vi "GenTargetSquat.vi"() -> ()   [LabVIEW 2016]
uses:
  Classes/CAlex2/TypeDef/CAlexVersion.ctl
  Sim&Process/DataProcess/CAlex2-Data/CAlex2_Data.lvclass
  C:/Users/Rand/Desktop/Bilateral-controller/CAlex2-controller/Sim&Process/DataProcess/ExpData/ExpData.lvclass
  Sim&Process/DataProcess/CAlex2-Data/PropertyNodes/Get_JointAngles.vi
  <vilib>/Utility/file.llb/Write Delimited Spreadsheet (string).vi
  <vilib>/Utility/file.llb/Write Delimited Spreadsheet (DBL).vi
  Sim&Process/DataProcess/ExpData/ExpData.lvclass
  <vilib>/AuZn/auzn custom VIs/AuZnCustomVI.lvlib
  Classes/CAlex2/CAlex2.lvclass
panel:
  out "TargetTraj 2":dbl[][](array[numeric])
  out "Xmin":dbl
  out "Xmax":dbl
  out "Ymin":dbl
  out "Ymax":dbl
  out "CAlexVersion":T1=enum."Mobile"
  out "AveragedJointAngle":dbl[][](array[numeric])
  out "TargetJointAngle":dbl[][](array[numeric])
  out "TargetTraj":dbl[][](array[numeric])
  in  "Save":bool
  in  "Ankle Flex":dbl=1.0 format="%#_13g"
  out "Leg Length":cluster{"Thigh":dbl, "Shank":dbl}
  in  "Scale Method":enum16{"Squat Depth", "Squat Angles"}(ring)
  in  "OutputLength":i32=500
  in  "Depth/Adduct":dbl=1.3 format="%#_13g"
  out "Array":dbl[](array[numeric])
  in  "Update":bool
  in  "Open":bool
  in  "stop":bool
  in  "EndTime":dbl=240.0
  in  "StartTime":dbl=60.0
  in  "Cut":bool
  out "AveragedTrajectory":dbl[][](graph)
  out "Averaged":cluster{"Mean":dbl[], "Mean":dbl[]}[](graph)
  out "Stacked":T2(graph)
  out "Ankle - X":dbl[][](graph)
  in  "Cut Parameter":dbl=100.0
  in  "Path":path=path "C:/Users/Rand/Desktop/squat simulated.txt"
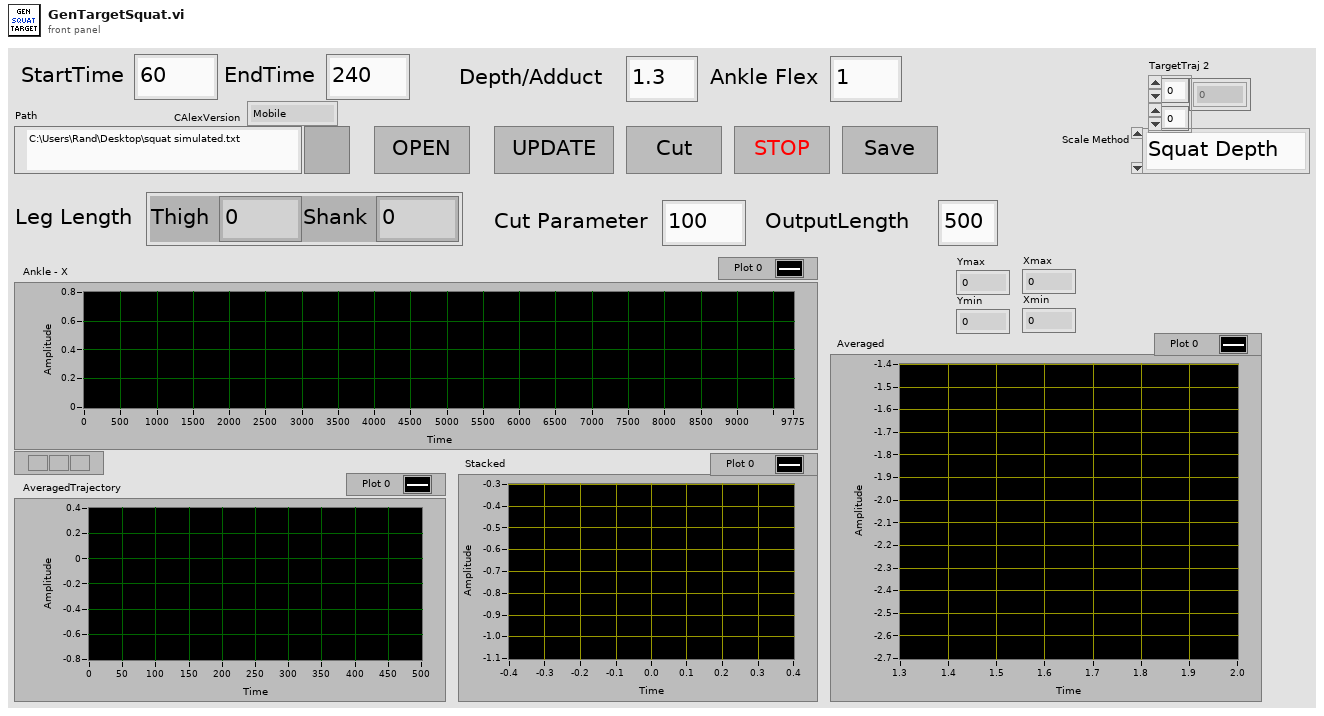
[diagram p1: front panel]
types:
  T1 = typedef "CAlex2.lvclass/CAlexVersion.ctl" = enum16{"Bilateral_Squat", "Squat", "Treadmill", "Mobile"}
  T2 = cluster{"DataAccess:WaistPosition":dbl[], "DataAccess:WaistPosition":dbl[]}
  T3 = enum16{"open", "replace", "create", "open or create", "replace or create", "replace or create with confirmation"}
  T4 = cluster{"ThighLt":dbl, "ShankLt":dbl, "HipWd":dbl}
  T5 = cluster{"ScaledJointAngles":dbl[], "ScaledJointAngles":dbl[]}
  T6 = cluster{"ScaledJointAngles":dbl[], "ScaledJointAngles":dbl[]}[]
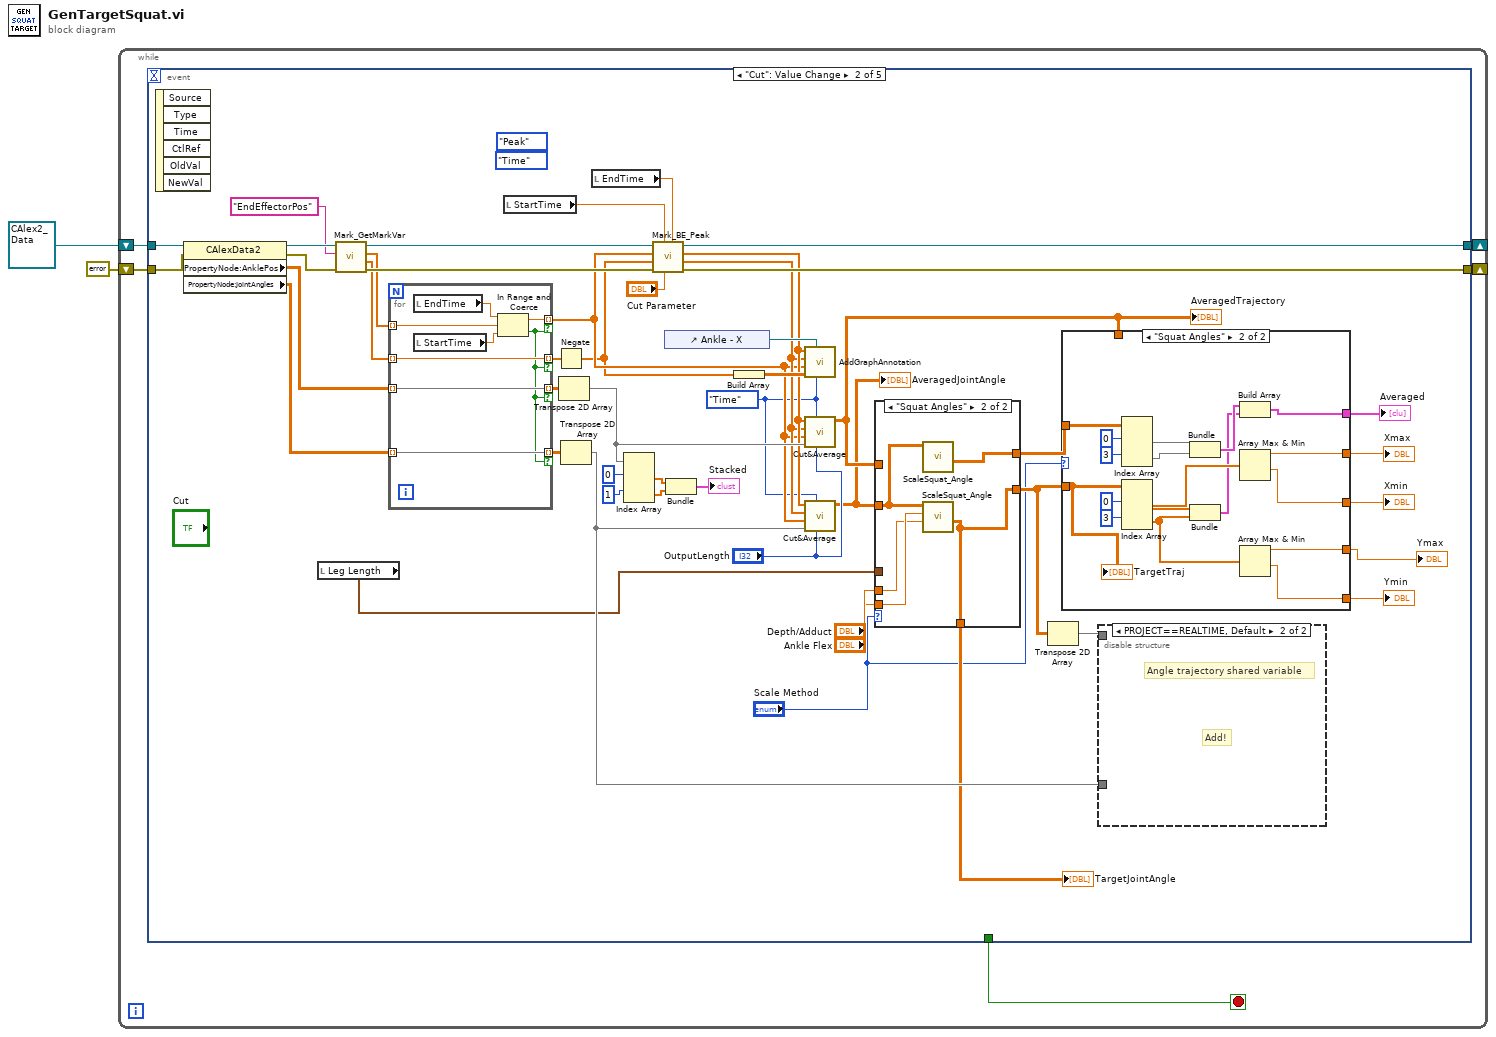
[diagram p0: block diagram]
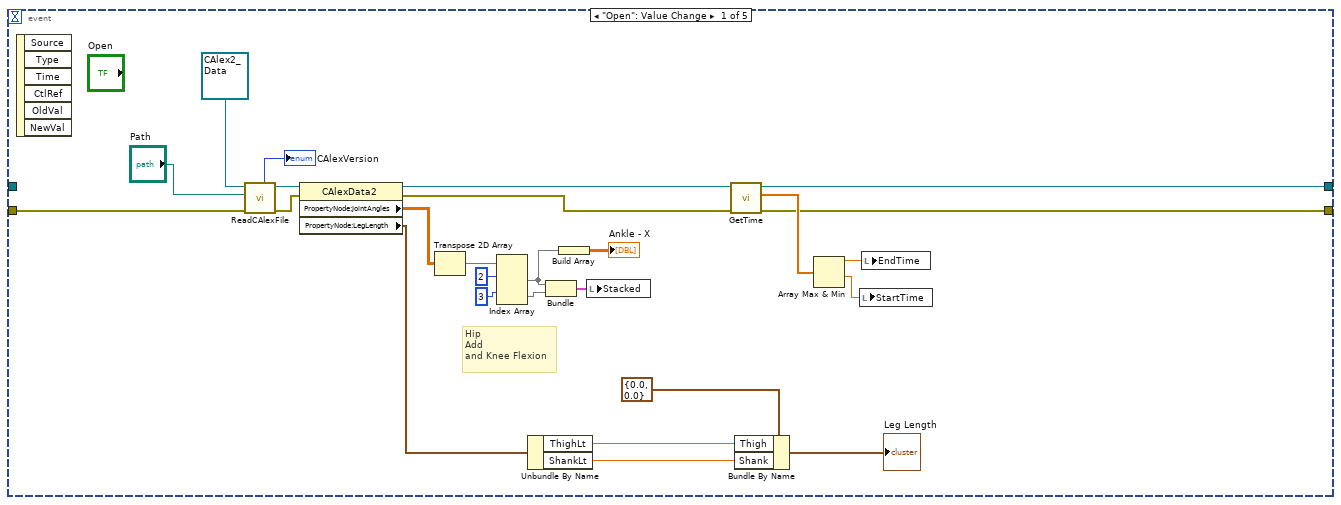
[diagram p2: hidden frame]
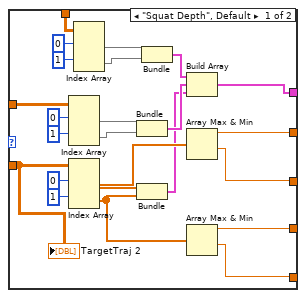
[diagram p3: hidden frame]
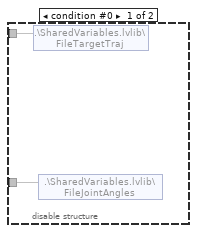
[diagram p4: hidden frame]
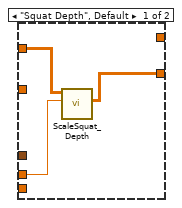
[diagram p5: hidden frame]
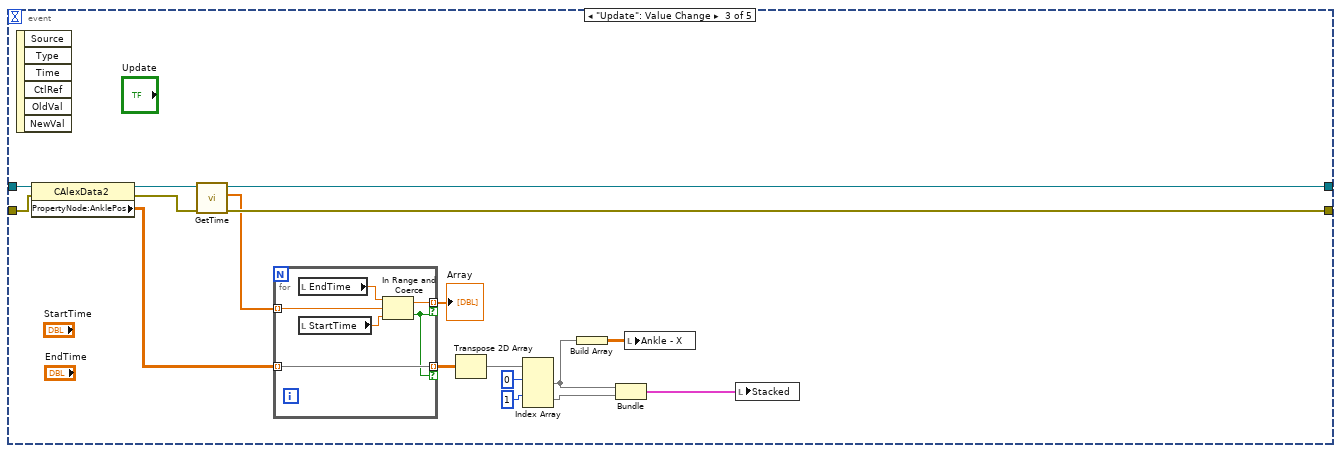
[diagram p6: hidden frame]
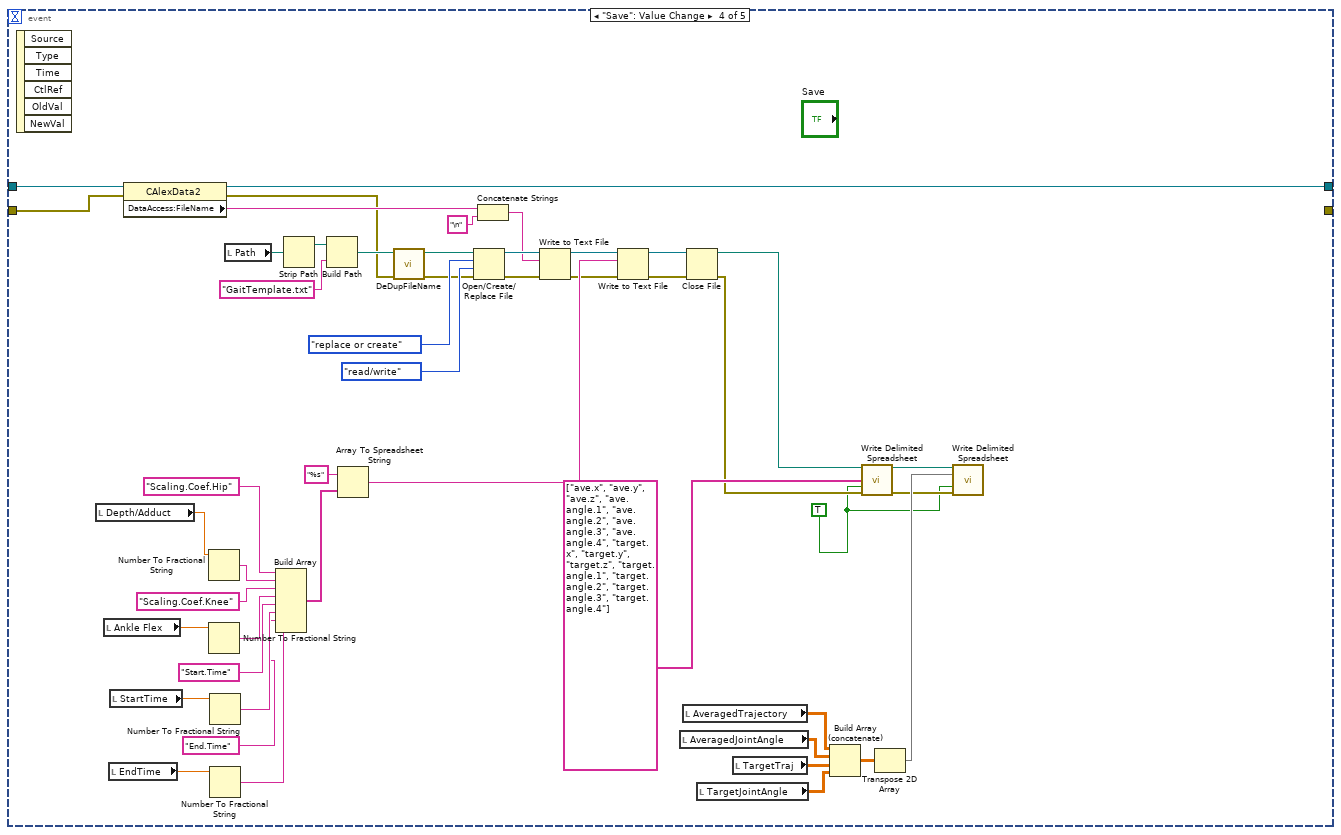
[diagram p7: hidden frame]
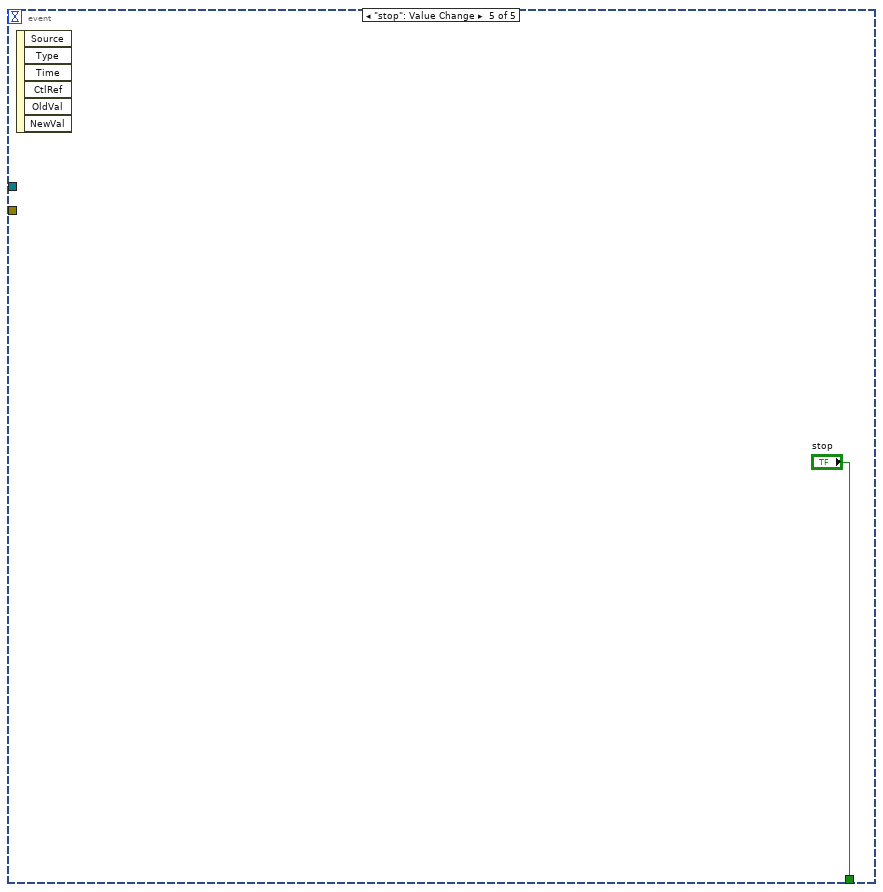
[diagram p8: hidden frame]
diagram:
  n1 = while {
    shift-right: [w4] -> _
    shift-left: refnum<class "CAlex2_Data.lvclass"> refnum ("CAlexData") -> [w7]
    shift-right: [w5] -> _
    shift-left: errorcluster {"status"=FALSE, "code"=0, "source"=""} ("error out") -> [w6]
    stop <- w3 stop-if-true
    n2 = event shown="[1] \"Cut\": Value Change" {
      selector: _ -> [_ _ _ _ _]
      dyn-events: _ -> [_ _ _ _ _]
      timeout: _ -> [_ _ _ _ _]
      tunnel: w7 -> [_ w74 w154 w176 _]
      tunnel: w6 -> [w23 w72 w153 w177 _]
      tunnel: [w20 w64 w145 _ _] -> w5
      tunnel: [w22 w63 w147 w175 _] -> w4
      tunnel: [_ _ _ _ "stop"] -> w3
      event "Open": Value Change {
        # "Hip\nAdd\nand Knee Flexion"
        n3 = event-data() -> ()  [unwired: 1 in, 6 out]
        n4 = call "ReadCAlexFile.vi"("error in (no error)"=w23, "ExpData File Path"="Path", "CAlexData2"=refnum<class "CAlex2_Data.lvclass"> refnum ("CAlexData")) -> ("error out"=w17:errorcluster, "CAlexData 2"=w19:refnum<class "CAlex2_Data.lvclass">, "CAlexVersion"=→"CAlexVersion":T1)  [unwired: 6 in]
        n5 = property class="CAlexData2"(reference=w19, error in=w17) -> (reference out=w18:refnum<class "CAlex2_Data.lvclass">, error out=w16:errorcluster, "PropertyNode:JointAngles"=w15:dbl[][], "PropertyNode:LegLength"=w14:T4)
        n6 = Transpose 2D Array(2D array=w15) -> (transposed array=w9:dbl[][])
        n7 = Index Array(array=w9, index (row) #1=2 ("index (row)"), index (row) #2=3 ("index (row)")) -> (element #1=w27:dbl[], element #2=w26:dbl[])  [unwired: 2 in]
        n8 = Unbundle By Name(w14) -> ("ThighLt"=w12:dbl, "ShankLt"=w11:dbl)
        n9 = Bundle(w27, w26) -> (w29:cluster{dbl[], dbl[]})  [unwired: 1 in]
        n10 = Build Array(w27) -> (→"Ankle - X":dbl[][])
        n11 = local write "Stacked"(w29) -> ()
        n12 = call "GetTime.vi"("error in (no error)"=w16, "ExpData in"=w18) -> ("error out"=w20:errorcluster, "Time"=w21:dbl[], "ExpData out"=w22:refnum<class "CAlex2_Data.lvclass">)  [unwired: 7 in]
        n13 = Bundle By Name(cluster=cluster{"Thigh":dbl, "Shank":dbl} {"Thigh"=0.0, "Shank"=0.0} ("Leg Length"), "Thigh"=w12, "Shank"=w11) -> (→"Leg Length":cluster{"Thigh":dbl, "Shank":dbl})
        n14 = Array Max & Min(array=w21) -> (max value=w33:dbl, min value=w32:dbl)  [unwired: 2 out]
        n15 = local write "StartTime"(w32) -> ()
        n16 = local write "EndTime"(w33) -> ()
      }
      event "Cut": Value Change {
        w57 = enum16{"Time", "Percentage", "Index"}."Time" ("Input Type")
        (unwired) enum16{"Peak", "Valley"}."Peak" ("Peak/Valley")
        (unwired) enum16{"Time", "Percentage", "Index"}."Time" ("Output Type")
        n17 = event-data() -> ()  [unwired: 1 in, 6 out]
        n18 = property class="CAlexData2"(reference=w74, error in=w72) -> (reference out=w73:refnum<class "CAlex2_Data.lvclass">, error out=w71:errorcluster, "PropertyNode:AnklePos"=w45:dbl[][], "PropertyNode:JointAngles"=w44:dbl[][])
        n19 = local read "Leg Length"() -> (w47:cluster{"Thigh":dbl, "Shank":dbl})
        n20 = call "Mark_GetMarkVar.vi"("error in (no error)"=w71, "VarName"="EndEffectorPos", "ExpData in"=w73) -> ("error out"=w81:errorcluster, "MarkVar"=w79:dbl[], "Time"=w80:dbl[], "ExpData out"=w75:refnum<class "CAlex2_Data.lvclass">)  [unwired: 3 in, 2 out]
        n21 = for {
          tunnel: w80 -> [w140] mode=indexing
          tunnel: w79 -> [w136] mode=indexing
          tunnel: [w137] -> w59 mode=indexing if=w133
          tunnel: [w136] -> w78 mode=indexing if=w133
          tunnel: w45 -> [w135] mode=indexing
          tunnel: [w135] -> w70 mode=indexing if=w133
          tunnel: w44 -> [w134] mode=indexing
          tunnel: [w134] -> w56 mode=indexing if=w133
          n22 = local read "EndTime"() -> (w138:dbl)
          n23 = local read "StartTime"() -> (w139:dbl)
          n24 = In Range and Coerce(upper limit=w138, x=w140, lower limit=w139) -> (coerced(x)=w137:dbl, In Range?=w133:bool)
        }
        n25 = local read "StartTime"() -> (w42:dbl)
        n26 = Negate(x=w78) -> (-x=w41:dbl[])
        n27 = Transpose 2D Array(2D array=w70) -> (transposed array=w62:dbl[][])
        n28 = Transpose 2D Array(2D array=w56) -> (transposed array=w51:dbl[][])
        n29 = local read "EndTime"() -> (w43:dbl)
        n30 = Index Array(array=w62, index (row) #1=0 ("index (row)"), index (row) #2=1 ("index (row)")) -> (element #1=w67:dbl[], element #2=w66:dbl[])  [unwired: 2 in]
        n31 = call "Mark_BE_Peak.vi"("End Time"=w43, "HalfWidth"="Cut Parameter", "Start Time"=w42, "error in (no error)"=w81, "Input"=w41, "Time"=w59, "CarexData In"=w75) -> ("error out"=w64:errorcluster, "End"=w60:dbl[], "Begin"=w61:dbl[], "CarexData Out"=w63:refnum<class "CAlex2_Data.lvclass">)  [unwired: 1 in]
        n32 = control-ref of="Ankle - X"() -> (w76:refnum<vi>)
        n33 = Bundle(w67, w66) -> (→"Stacked":cluster{dbl[], dbl[]})  [unwired: 1 in]
        n34 = Build Array(w41) -> (w77:dbl[][])
        n35 = call <vilib>:"AddGraphAnnotation.vi"("Input Type (Time)"=w57, "WaveformGraph in"=w76, "Array"=w77, "Time"=w59, "Valleys  (Yellow)"=w60, "Peaks (Red)"=w61) -> ()  [unwired: 4 in, 2 out]
        n36 = call <vilib>:"Cut&Average.vi"("Dilate Length (200)"="OutputLength", "Input Type (Time)"=w57, "Data"=w62, "Time"=w59, "End"=w60, "Begin"=w61) -> ("Mean"=w54:dbl[][])  [unwired: 5 out]
        "AveragedTrajectory" <- w54
        n37 = call <vilib>:"Cut&Average.vi"("Dilate Length (200)"="OutputLength", "Input Type (Time)"=w57, "Data"=w51, "Time"=w59, "End"=w60, "Begin"=w61) -> ("Mean"=w50:dbl[][])  [unwired: 5 out]
        "AveragedJointAngle" <- w50
        n38 = case shown="\"Squat Angles\"" "Scale Method" {
          tunnel: [w126 w130] -> w52
          tunnel: w50 -> [_ w132]
          tunnel: w47 -> [_ _]
          tunnel: "Depth/Adduct" -> [w127 w128]
          tunnel: w54 -> [w125 _]
          tunnel: "Ankle Flex" -> [_ w129]
          tunnel: [_ w130] -> w49
          tunnel: [_ w131] -> w48
          frame "Squat Depth", Default {
            n39 = call "ScaleSquat_Depth.vi"("ScalingCoef"=w127, "Averaged Squat Trajectory"=w125) -> ("ScaledGait"=w126:dbl[][])  [unwired: 8 in, 1 out]
          }
          frame "Squat Angles" {
            n40 = call "ScaleSquat_Angle.vi"("AverageJointAngles"=w132) -> ("ScaledJointAngles"=w131:dbl[][])  [unwired: 10 in]
            n41 = call "ScaleSquat_Angle.vi"("ScalingCoef Hip Add"=w128, "ScalingCoef Ankle Flex"=w129, "AverageJointAngles"=w132) -> ("ScaledJointAngles"=w130:dbl[][])  [unwired: 8 in]
          }
        }
        "TargetJointAngle" <- w49
        n42 = Transpose 2D Array(2D array=w52) -> (transposed array=w40:dbl[][])
        n43 = case shown="\"Squat Angles\"" "Scale Method" {
          tunnel: w54 -> [w99 _]
          tunnel: w52 -> [w98 w120]
          tunnel: w48 -> [w93 w115]
          tunnel: [w84 w110] -> w38
          tunnel: [w85 w109] -> w37
          tunnel: [w86 w108] -> w34
          tunnel: [w87 w107] -> w36
          tunnel: [w83 w106] -> w35
          frame "Squat Depth", Default {
            n44 = Index Array(array=w93, index (row) #1=0 ("index (row)"), index (row) #2=1 ("index (row)")) -> (element #1=w95:dbl[], element #2=w94:dbl[])  [unwired: 2 in]
            n45 = Index Array(array=w98, index (row) #1=0 ("index (row)"), index (row) #2=1 ("index (row)")) -> (element #1=w89:dbl[], element #2=w90:dbl[])  [unwired: 2 in]
            n46 = Index Array(array=w99, index (row) #1=0 ("index (row)"), index (row) #2=1 ("index (row)")) -> (element #1=w102:dbl[], element #2=w103:dbl[])  [unwired: 2 in]
            n47 = Bundle("ScaledJointAngles"=w95, "ScaledJointAngles"=w94) -> (w91:T5)  [unwired: 1 in]
            n48 = Bundle("ScaledJointAngles"=w89, "ScaledJointAngles"=w90) -> (w88:T5)  [unwired: 1 in]
            n49 = Bundle("Mean"=w102, "Mean"=w103) -> (w92:cluster{"Mean":dbl[], "Mean":dbl[]})  [unwired: 1 in]
            n50 = Build Array(w92, w91, w88) -> (w83:T6)
            n51 = Array Max & Min(array=w89) -> (max value=w84:dbl, min value=w85:dbl)  [unwired: 2 out]
            n52 = Array Max & Min(array=w90) -> (max value=w86:dbl, min value=w87:dbl)  [unwired: 2 out]
            "TargetTraj 2" <- w98
          }
          frame "Squat Angles" {
            n53 = Index Array(array=w115, index (row) #1=0 ("index (row)"), index (row) #2=3 ("index (row)")) -> (element #1=w117:dbl[], element #2=w116:dbl[])  [unwired: 2 in]
            n54 = Index Array(array=w120, index (row) #1=0 ("index (row)"), index (row) #2=3 ("index (row)")) -> (element #1=w112:dbl[], element #2=w113:dbl[])  [unwired: 2 in]
            n55 = Bundle("ScaledJointAngles"=w117, "ScaledJointAngles"=w116) -> (w114:T5)  [unwired: 1 in]
            n56 = Bundle("ScaledJointAngles"=w112, "ScaledJointAngles"=w113) -> (w111:T5)  [unwired: 1 in]
            n57 = Build Array(w114, w111) -> (w106:T6)
            n58 = Array Max & Min(array=w112) -> (max value=w110:dbl, min value=w109:dbl)  [unwired: 2 out]
            n59 = Array Max & Min(array=w113) -> (max value=w108:dbl, min value=w107:dbl)  [unwired: 2 out]
            "TargetTraj" <- w120
          }
        }
        "Ymax" <- w34
        "Ymin" <- w36
        "Xmax" <- w38
        "Xmin" <- w37
        "Averaged" <- w35
        n60 = disable-structure shown="PROJECT==REALTIME, Default" {
          disable-tunnel: w40 -> [w124 _]
          disable-tunnel: w51 -> [w123 _]
          frame condition #0 {
            n61 = shared-variable ".\\SharedVariables.lvlib\\FileTargetTraj"(w124) -> ()  [unwired: 1 in, 1 out]
            n62 = shared-variable ".\\SharedVariables.lvlib\\FileJointAngles"(w123) -> ()  [unwired: 1 in, 1 out]
          }
          frame condition #1 (active) {
            # "Add!"
            # "Angle trajectory shared variable"
          }
        }
      }
      event "Update": Value Change {
        n63 = event-data() -> ()  [unwired: 1 in, 6 out]
        n64 = property class="CAlexData2"(reference=w154, error in=w153) -> (reference out=w148:refnum<class "CAlex2_Data.lvclass">, error out=w146:errorcluster, "PropertyNode:AnklePos"=w143:dbl[][])
        n65 = call "GetTime.vi"("error in (no error)"=w146, "ExpData in"=w148) -> ("error out"=w145:errorcluster, "Time"=w144:dbl[], "ExpData out"=w147:refnum<class "CAlex2_Data.lvclass">)  [unwired: 7 in]
        n66 = for {
          tunnel: w144 -> [w163] mode=indexing
          tunnel: [w160] -> w152 mode=indexing if=w158
          tunnel: w143 -> [w159] mode=indexing
          tunnel: [w159] -> w142 mode=indexing if=w158
          n67 = local read "EndTime"() -> (w161:dbl)
          n68 = local read "StartTime"() -> (w162:dbl)
          n69 = In Range and Coerce(upper limit=w161, x=w163, lower limit=w162) -> (coerced(x)=w160:dbl, In Range?=w158:bool)
        }
        "Array" <- w152
        n70 = Transpose 2D Array(2D array=w142) -> (transposed array=w141:dbl[][])
        n71 = Index Array(array=w141, index (row) #1=0 ("index (row)"), index (row) #2=1 ("index (row)")) -> (element #1=w150:dbl[], element #2=w149:dbl[])  [unwired: 2 in]
        n72 = Build Array(w150) -> (w151:dbl[][])
        n73 = Bundle(w150, w149) -> (w155:cluster{dbl[], dbl[]})  [unwired: 1 in]
        n74 = local write "Ankle - X"(w151) -> ()
        n75 = local write "Stacked"(w155) -> ()
      }
      event "Save": Value Change {
        w164 = TRUE ("append to file? (new file:F)")
        n76 = event-data() -> ()  [unwired: 1 in, 6 out]
        n77 = local read "Depth/Adduct"() -> (w203:dbl)
        n78 = local read "Ankle Flex"() -> (w202:dbl)
        n79 = local read "EndTime"() -> (w187:dbl)
        n80 = local read "StartTime"() -> (w186:dbl)
        n81 = property class="CAlexData2"(reference=w176, error in=w177) -> (reference out=w175:refnum<class "CAlex2_Data.lvclass">, error out=w165:errorcluster, "DataAccess:FileName"=w174:string)
        n82 = Number To Fractional String(number=w203) -> (F-format string=w200:string)  [unwired: 3 in]
        n83 = Number To Fractional String(number=w202) -> (F-format string=w198:string)  [unwired: 3 in]
        n84 = Number To Fractional String(number=w186) -> (F-format string=w184:string)  [unwired: 3 in]
        n85 = Number To Fractional String(number=w187) -> (F-format string=w182:string)  [unwired: 3 in]
        n86 = local read "Path"() -> (w211:path)
        n87 = Build Array("Scaling.Coef.Hip" ("name or relative path"), w200, "Scaling.Coef.Knee" ("name or relative path"), w198, "Start.Time" ("name or relative path"), w184, "End.Time" ("name or relative path"), w182) -> (w197:string[])
        n88 = Strip Path(path=w211) -> (stripped path=w209:path)  [unwired: 1 out]
        n89 = Build Path(base path=w209, name or relative path="GaitTemplate.txt") -> (appended path=w168:path)
        n90 = Array To Spreadsheet String(array=w197, 3:"%s" ("format string")) -> (spreadsheet string=w196:string)  [unwired: 1 in]
        n91 = call <vilib>:"DeDupFileName.vi"("error in (no error)"=w165, "Path"=w168) -> ("error out"=w166:errorcluster, "Out Path"=w167:path)  [unwired: 7 in, 1 out]
        n92 = Open/Create/Replace File(file path (use dialog)=w167, error in=w166, operation (0:open)=T3."replace or create", access (0:read/write)=enum16{"read/write", "read-only", "write-only"}."read/write") -> (refnum out=w181:refnum<file>, error out=w179:errorcluster)  [unwired: 2 in, 1 out]
        n93 = Concatenate Strings(w174, "\n" ("string")) -> (w173:string)
        n94 = Write to Text File(file (use dialog)=w181, text=w173, error in=w179) -> (refnum out=w180:refnum<file>, error out=w178:errorcluster)  [unwired: 1 in, 1 out]
        n95 = Write to Text File(file (use dialog)=w180, text=w196, error in=w178) -> (refnum out=w192:refnum<file>, error out=w193:errorcluster)  [unwired: 1 in, 1 out]
        n96 = local read "AveragedJointAngle"() -> (w189:dbl[][])
        n97 = local read "AveragedTrajectory"() -> (w190:dbl[][])
        n98 = Close File(refnum=w192, error in=w193) -> (path=w191:path, error out=w170:errorcluster)
        n99 = local read "TargetJointAngle"() -> (w207:dbl[][])
        n100 = local read "TargetTraj"() -> (w210:dbl[][])
        n101 = Build Array (concatenate)(w190, w189, w210, w207) -> (w206:dbl[][])
        n102 = call-poly <vilib>:"Write Delimited Spreadsheet.vi"("file path (dialog if empty)"=w191, "1D data"=string[] ["ave.x", "ave.y", "ave.z", "ave.angle.1", "ave.angle.2", "ave.angle.3", "ave.angle.4", "target.x", "target.y", "target.z", "target.angle.1", "target.angle.2", "target.angle.3", "target.angle.4"], "append to file? (new file:F)"=w164, "error in (no error)"=w170) -> ("new file path (Not A Path if cancelled)"=w205:path, "error out"=w169:errorcluster)  [unwired: 10 in]
        n103 = Transpose 2D Array(2D array=w206) -> (transposed array=w204:dbl[][])
        n104 = call-poly <vilib>:"Write Delimited Spreadsheet.vi"("file path (dialog if empty)"=w205, "2D data"=w204, "append to file? (new file:F)"=w164, "error in (no error)"=w169) -> ()  [unwired: 10 in, 2 out]
      }
      event "stop": Value Change {
        n105 = event-data() -> ()  [unwired: 1 in, 6 out]
      }
    }
  }
